vi "Convert Endpoint to UI Element.vi"(11 "Connection":T1) -> (3 "Channel":T3)   [LabVIEW 2019, in "NI-SWITCH System Explorer.lvlib"]
uses:
  NI-SWITCH System Explorer.lvlib
  Channel.ctl
  Channel Type.ctl
  Shared/Endpoint Configuration Cluster.ctl
  Shared/Endpoint Configuration Enum.ctl
  Shared/NI-SWITCH Shared.lvlib
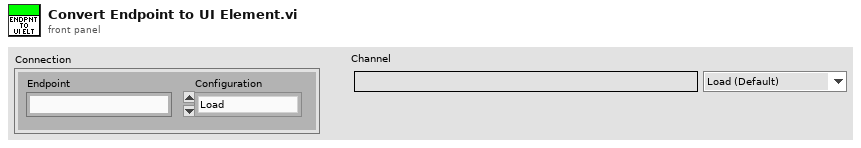
[diagram p1: front panel]
types:
  T1 = typedef "NI-SWITCH Shared.lvlib/Endpoint Configuration Cluster.ctl" = cluster{"Endpoint":string, "Configuration":T2}
  T2 = typedef "NI-SWITCH Shared.lvlib/Endpoint Configuration Enum.ctl" = enum16{"Load", "Source", "Configuration"}
  T3 = typedef "NI-SWITCH System Explorer.lvlib/Channel.ctl" = cluster{"Endpoint":string, "Configuration":T4}
  T4 = typedef "NI-SWITCH System Explorer.lvlib/Channel Type.ctl" = enum16{"Load (Default)", "Source", "Configuration"}
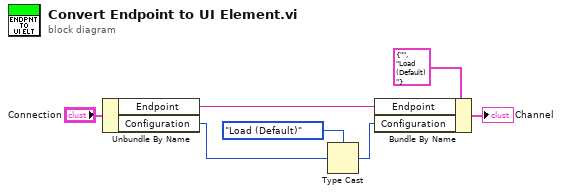
[diagram p0: block diagram]
diagram:
  n1 = Unbundle By Name("Connection") -> ("Endpoint"=w1:string, "Configuration"=w4:T2)
  n2 = Type Cast(type=Channel_Type."Load (Default)" ("Alias"), x=w4) -> (*(type *) &x=w6:T4)
  n3 = Bundle By Name(cluster=T3 {"Endpoint"="", "Configuration"=enum."Load (Default)"} ("Channel"), "Endpoint"=w1, "Configuration"=w6) -> (→"Channel":T3)
